vi "Reset Wait.vi"(8 "error in":errorcluster, 10 "Time to Reset(ms) (2min)":u32=120000, 11 "VISA resource name":refnum<visa-resource-name>) -> (0 "error out":errorcluster, 2 "Comm OK?":bool, 3 "VISA resource name out":refnum<visa-resource-name>)   [LabVIEW 2009, in "Digikrom DK24x.lvlib"]
doc: "Waits for the monochromator to come back online (after a reset or reboot operation) by pinging it every two seconds."
uses:
  Digikrom DK24x.lvlib
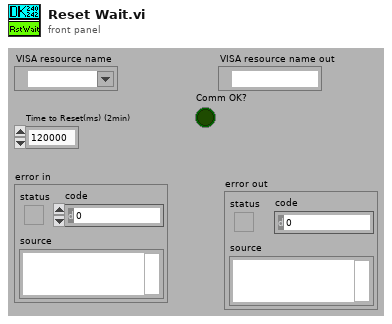
[diagram p1: front panel]
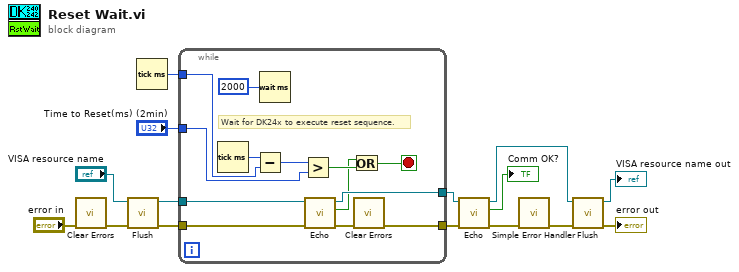
[diagram p0: block diagram]
diagram:
  n1 = call <vilib>:"Clear Errors.vi"("error in (no error)"="error in") -> ("error out"=w3:errorcluster)  [unwired: 6 out]
  n2 = call "Flush.vi"("error in (no error)"=w3, "VISA resource name"="VISA resource name") -> ("error out"=w2:errorcluster, "VISA resource name out"=w4:refnum<visa-resource-name>)  [unwired: 8 out]
  n3 = Tick Count (ms)() -> (millisecond timer value=w7:u32)
  n4 = while {
    tunnel: "Time to Reset(ms) (2min)" -> [w27]
    tunnel: [w26] -> w13
    tunnel: w4 -> [w25]
    tunnel: w7 -> [w20]
    tunnel: [w18] -> w12
    tunnel: w2 -> [w16]
    stop <- w28 stop-if-true
    # "Wait for DK24x to execute reset sequence."
    n5 = Tick Count (ms)() -> (millisecond timer value=w22:u32)
    n6 = Subtract(x=w22, y=w20) -> (x-y=w23:u32)
    n7 = Wait (ms)(milliseconds to wait=u32 2000) -> ()  [unwired: 1 out]
    n8 = Greater?(x=w23, y=w27) -> (0:w24:bool)
    n9 = call "Echo.vi"("error in (no error)"=w16, "VISA resource name"=w25) -> ("error out"=w19:errorcluster, "Comm OK?"=w21:bool, "VISA resource name out"=w26:refnum<visa-resource-name>)  [unwired: 7 out]
    n10 = Or(x=w21, y=w24) -> (x .or. y?=w28:bool)
    n11 = call <vilib>:"Clear Errors.vi"("error in (no error)"=w19) -> ("error out"=w18:errorcluster)  [unwired: 6 out]
  }
  n12 = call "Echo.vi"("error in (no error)"=w12, "VISA resource name"=w13) -> ("error out"=w10:errorcluster, "Comm OK?"=→"Comm OK?":bool, "VISA resource name out"=w11:refnum<visa-resource-name>)  [unwired: 7 out]
  n13 = call <vilib>:"Simple Error Handler.vi"("error in (no error)"=w10) -> ("error out"=w9:errorcluster)  [unwired: 1 in, 7 out]
  n14 = call "Flush.vi"("error in (no error)"=w9, "VISA resource name"=w11) -> ("error out"=→"error out":errorcluster, "VISA resource name out"=→"VISA resource name out":refnum<visa-resource-name>)  [unwired: 8 out]
